vi "dfd_Combine Single Orders.vi"(1 "P(z) in":cluster{"Ni(z)":dbl[]}[](array[cluster])=[{"Ni(z)"=[1.0]}, {"Ni(z)"=[1.0, 1.0]}, {"Ni(z)"=[1.0, 1.0]}, {"Ni(z)"=[1.0, 1.0]}, {"Ni(z)"=[1.0, 1.0]}, {"Ni(z)"=[1.0, 1.0]}, {"Ni(z)"=[1.0, 1.0]}] {"Ni(z)" format="%.2f"}) -> (0 "P(z) out":cluster{"Ni(z)":dbl[]}[](array[cluster])=[{"Ni(z)"=[1.0]}, {"Ni(z)"=[1.0, 1.0]}, {"Ni(z)"=[1.0, 1.0]}, {"Ni(z)"=[1.0, 1.0]}, {"Ni(z)"=[1.0, 1.0]}, {"Ni(z)"=[1.0, 1.0]}, {"Ni(z)"=[1.0, 1.0]}] {"Ni(z)" format="%.2f"})   [LabVIEW 2017, in "NI_DigFilter_Design.lvlib"]
uses:
  <vilib>/addons/Digital Filter Design/NI_DigFilter_Design.lvlib
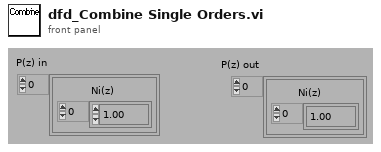
[diagram p1: front panel]
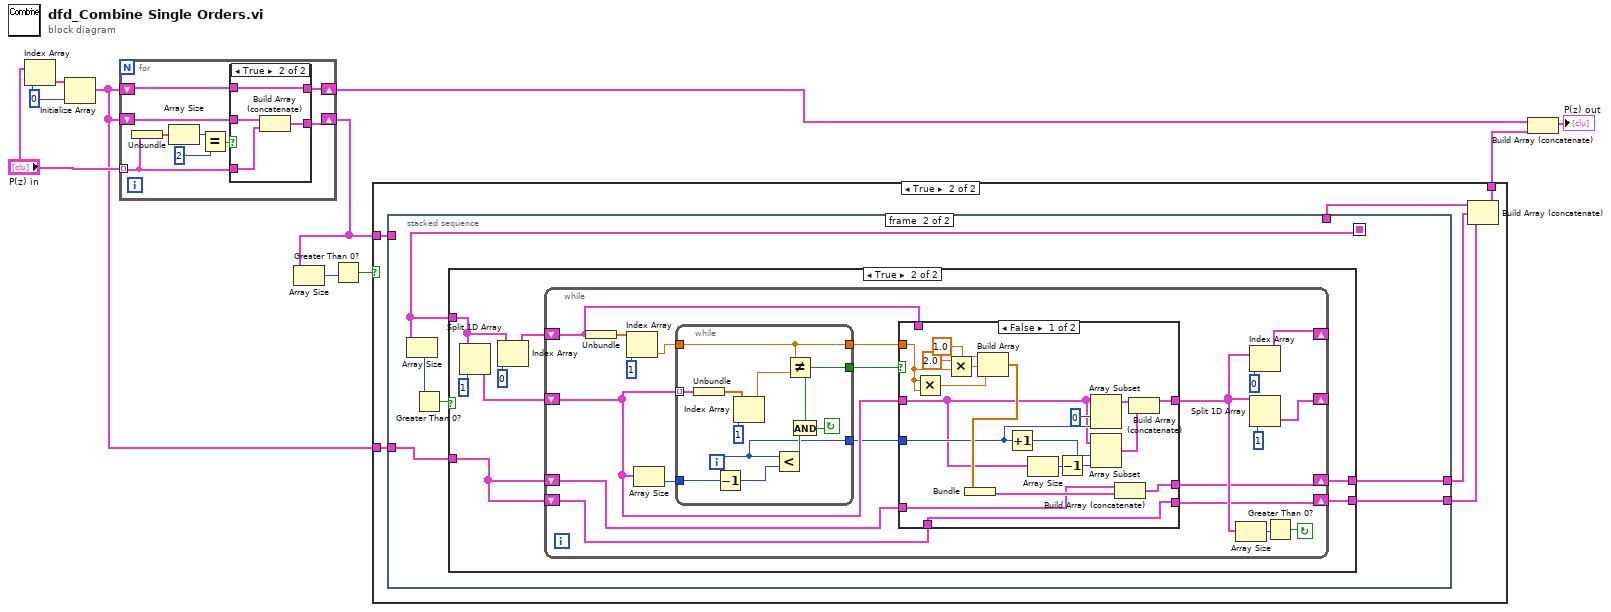
[diagram p0: block diagram]
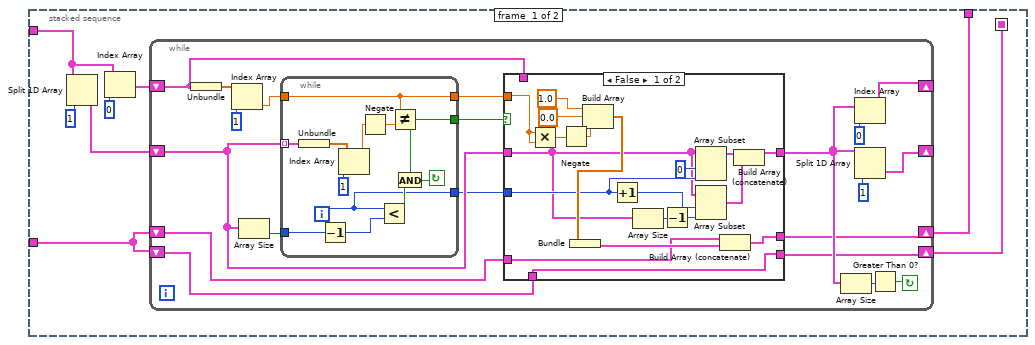
[diagram p3: hidden frame]
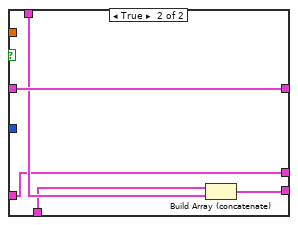
[diagram p4: hidden frame]
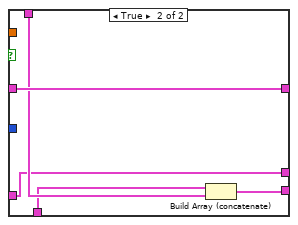
[diagram p6: hidden frame]
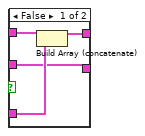
[diagram p7: hidden frame]
diagram:
  w8 = 0
  n1 = Index Array(array="P(z) in", index=w8) -> (element=w9:cluster{"Ni(z)":dbl[]})
  n2 = Initialize Array(w9, w8) -> (w2:cluster{"Ni(z)":dbl[]}[])
  n3 = for {
    shift-right: [w14] -> w7
    shift-left: w2 -> [w13]
    tunnel: "P(z) in" -> [w15] mode=indexing
    shift-right: [w12] -> w3
    shift-left: w2 -> [w11]
    n4 = Unbundle(w15) -> ("Ni(z)"=w19:dbl[])
    n5 = Array Size(array=w19) -> (size(s)=w16:i32)
    n6 = Equal?(x=w16, y=2) -> (x = y?=w18:bool)
    n7 = case shown="True" w18 {
      tunnel: w15 -> [w23 w27]
      tunnel: w13 -> [w21 w24]
      tunnel: [w22 w24] -> w14
      tunnel: [w20 w26] -> w12
      tunnel: w11 -> [w20 w25]
      frame False {
        n8 = Build Array (concatenate)(w21, w23) -> (w22:cluster{"Ni(z)":dbl[]}[])
      }
      frame True {
        n9 = Build Array (concatenate)(w25, w27) -> (w26:cluster{"Ni(z)":dbl[]}[])
      }
    }
  }
  n10 = Array Size(array=w3) -> (size(s)=w5:i32)
  n11 = Greater Than 0?(x=w5) -> (x > 0?=w4:bool)
  n12 = case shown="True" w4 {
    tunnel: w3 -> [_ w34]
    tunnel: [w28 w32] -> w1
    tunnel: w2 -> [w28 w29]
    frame False {
    }
    frame True {
      n13 = stacked-sequence {
        seq-local: [w39 _] -> [_ w103]
        tunnel: w29 -> [w38 w99]
        tunnel: [w37 _] -> w33
        tunnel: w34 -> [w36 _]
        tunnel: [_ w101] -> w31
        tunnel: [_ w100] -> w30
        frame #0 {
          n14 = Split 1D Array(array=w36, index=1) -> (second subarray=w42:cluster{"Ni(z)":dbl[]}[])  [unwired: 1 out]
          n15 = Index Array(array=w36, index=0) -> (element=w35:cluster{"Ni(z)":dbl[]})
          n16 = while {
            shift-left: w38 -> [w46]
            shift-right: [w44] -> w39
            shift-left: w42 -> [w55]
            shift-right: [w49] -> _
            shift-left: w35 -> [w56]
            shift-right: [w51] -> _
            shift-left: w38 -> [w47]
            shift-right: [w45] -> w37
            stop <- w43 continue-if-true
            n17 = Unbundle(w56) -> ("Ni(z)"=w58:dbl[])
            n18 = Index Array(array=w58, index=1) -> (element=w60:dbl)
            n19 = Array Size(array=w55) -> (size(s)=w61:i32)
            n20 = while {
              tunnel: [w64] -> w54
              tunnel: [w65] -> w57
              tunnel: [w68] -> w59
              tunnel: w60 -> [w65]
              tunnel: w61 -> [w72]
              tunnel: w55 -> [w73] mode=indexing
              i -> [w64]
              stop <- w67 continue-if-true
              n21 = Unbundle(w73) -> ("Ni(z)"=w66:dbl[])
              n22 = Decrement(x=w72) -> (x-1=w63:i32)
              n23 = Index Array(array=w66, index=1) -> (element=w71:dbl)
              n24 = Negate(x=w71) -> (-x=w70:dbl)
              n25 = Less?(x=w64, y=w63) -> (x < y?=w69:bool)
              n26 = Not Equal?(x=w65, y=w70) -> (x != y?=w68:bool)
              n27 = And(x=w68, y=w69) -> (x .and. y?=w67:bool)
            }
            n28 = case shown="False" w59 {
              tunnel: w57 -> [w89 _]
              tunnel: w56 -> [_ w97]
              tunnel: w55 -> [w79 w98]
              tunnel: [w82 w98] -> w48
              tunnel: w54 -> [w87 _]
              tunnel: [w76 w95] -> w44
              tunnel: w47 -> [w77 w94]
              tunnel: w46 -> [w76 w96]
              tunnel: [w75 w94] -> w45
              frame False {
                n29 = Multiply(x=w89, y=w89) -> (x*y=w91:dbl)
                n30 = Negate(x=w91) -> (-x=w90:dbl)
                n31 = Build Array(1.0, 0.0, w90) -> (w88:dbl[])
                n32 = Bundle(w88) -> (w78:cluster{dbl[]})  [unwired: 1 in]
                n33 = Increment(x=w87) -> (x+1=w83:i32)
                n34 = Array Size(array=w79) -> (size(s)=w85:i32)
                n35 = Decrement(x=w85) -> (x-1=w84:i32)
                n36 = Array Subset(array=w79, index=0, length=w87) -> (w80:cluster{"Ni(z)":dbl[]}[])
                n37 = Array Subset(array=w79, index=w83, length=w84) -> (w81:cluster{"Ni(z)":dbl[]}[])
                n38 = Build Array (concatenate)(w77, w78) -> (w75:cluster{"Ni(z)":dbl[]}[])
                n39 = Build Array (concatenate)(w80, w81) -> (w82:cluster{"Ni(z)":dbl[]}[])
              }
              frame True {
                n40 = Build Array (concatenate)(w96, w97) -> (w95:cluster{"Ni(z)":dbl[]}[])
              }
            }
            n41 = Array Size(array=w48) -> (size(s)=w50:i32)
            n42 = Index Array(array=w48, index=0) -> (element=w51:cluster{"Ni(z)":dbl[]})
            n43 = Split 1D Array(array=w48, index=1) -> (second subarray=w49:cluster{"Ni(z)":dbl[]}[])  [unwired: 1 out]
            n44 = Greater Than 0?(x=w50) -> (x > 0?=w43:bool)
          }
        }
        frame #1 {
          n45 = Array Size(array=w103) -> (size(s)=w104:i32)
          n46 = Greater Than 0?(x=w104) -> (x > 0?=w102:bool)
          n47 = case shown="True" w102 {
            tunnel: w103 -> [_ w113]
            tunnel: [w105 w108] -> w101
            tunnel: [w105 w107] -> w100
            tunnel: w99 -> [w105 w106]
            frame False {
            }
            frame True {
              n48 = Split 1D Array(array=w113, index=1) -> (second subarray=w109:cluster{"Ni(z)":dbl[]}[])  [unwired: 1 out]
              n49 = Index Array(array=w113, index=0) -> (element=w110:cluster{"Ni(z)":dbl[]})
              n50 = while {
                shift-left: w106 -> [w117]
                shift-right: [w115] -> w107
                shift-left: w109 -> [w126]
                shift-right: [w120] -> _
                shift-left: w110 -> [w127]
                shift-right: [w122] -> _
                shift-left: w106 -> [w118]
                shift-right: [w116] -> w108
                stop <- w114 continue-if-true
                n51 = Unbundle(w127) -> ("Ni(z)"=w129:dbl[])
                n52 = Index Array(array=w129, index=1) -> (element=w131:dbl)
                n53 = Array Size(array=w126) -> (size(s)=w132:i32)
                n54 = while {
                  tunnel: [w136] -> w125
                  tunnel: [w137] -> w128
                  tunnel: [w140] -> w130
                  tunnel: w131 -> [w137]
                  tunnel: w132 -> [w142]
                  tunnel: w126 -> [w143] mode=indexing
                  i -> [w136]
                  stop <- w139 continue-if-true
                  n55 = Unbundle(w143) -> ("Ni(z)"=w138:dbl[])
                  n56 = Decrement(x=w142) -> (x-1=w135:i32)
                  n57 = Index Array(array=w138, index=1) -> (element=w134:dbl)
                  n58 = Less?(x=w136, y=w135) -> (x < y?=w141:bool)
                  n59 = Not Equal?(x=w137, y=w134) -> (x != y?=w140:bool)
                  n60 = And(x=w140, y=w141) -> (x .and. y?=w139:bool)
                }
                n61 = case shown="False" w130 {
                  tunnel: w128 -> [w146 _]
                  tunnel: w127 -> [_ w167]
                  tunnel: w126 -> [w152 w168]
                  tunnel: [w155 w168] -> w119
                  tunnel: w125 -> [w160 _]
                  tunnel: [w149 w165] -> w115
                  tunnel: w118 -> [w150 w164]
                  tunnel: w117 -> [w149 w166]
                  tunnel: [w148 w164] -> w116
                  frame False {
                    n62 = Multiply(x=w146, y=w146) -> (x*y=w162:dbl)
                    n63 = Multiply(x=2.0, y=w146) -> (x*y=w145:dbl)
                    n64 = Build Array(1.0, w145, w162) -> (w161:dbl[])
                    n65 = Bundle(w161) -> (w151:cluster{dbl[]})  [unwired: 1 in]
                    n66 = Increment(x=w160) -> (x+1=w156:i32)
                    n67 = Array Size(array=w152) -> (size(s)=w158:i32)
                    n68 = Decrement(x=w158) -> (x-1=w157:i32)
                    n69 = Array Subset(array=w152, index=0, length=w160) -> (w153:cluster{"Ni(z)":dbl[]}[])
                    n70 = Array Subset(array=w152, index=w156, length=w157) -> (w154:cluster{"Ni(z)":dbl[]}[])
                    n71 = Build Array (concatenate)(w150, w151) -> (w148:cluster{"Ni(z)":dbl[]}[])
                    n72 = Build Array (concatenate)(w153, w154) -> (w155:cluster{"Ni(z)":dbl[]}[])
                  }
                  frame True {
                    n73 = Build Array (concatenate)(w166, w167) -> (w165:cluster{"Ni(z)":dbl[]}[])
                  }
                }
                n74 = Array Size(array=w119) -> (size(s)=w121:i32)
                n75 = Index Array(array=w119, index=0) -> (element=w122:cluster{"Ni(z)":dbl[]})
                n76 = Split 1D Array(array=w119, index=1) -> (second subarray=w120:cluster{"Ni(z)":dbl[]}[])  [unwired: 1 out]
                n77 = Greater Than 0?(x=w121) -> (x > 0?=w114:bool)
              }
            }
          }
        }
      }
      n78 = Build Array (concatenate)(w33, w31, w30) -> (w32:cluster{"Ni(z)":dbl[]}[])
    }
  }
  n79 = Build Array (concatenate)(w7, w1) -> (→"P(z) out":cluster{"Ni(z)":dbl[]}[])
